vi "SA Configure.vi"(7 "RBW(Hz)":dbl=1.0, 8 "number of records":dbl=1.0, 9 "samples per record":dbl=100.0, 10 "IQ Rate (S/s)":dbl=4000000.0 format="%#.3p", 11 "Semiconductor Module Context":T1) -> (0 "error out":errorcluster)   [LabVIEW 2014]
uses:
  <vilib>/NI_TestStand_SemiconductorModule/NI_TestStand_Semiconductor_Module.lvlibp/PinMap/General/SemiconductorModuleContext.ctl
  <instrlib>/niRFSA/niRFSA.llb/niRFSA Acquisition Types.ctl
  <vilib>/NI_TestStand_SemiconductorModule/NI_TestStand_Semiconductor_Module.lvlibp
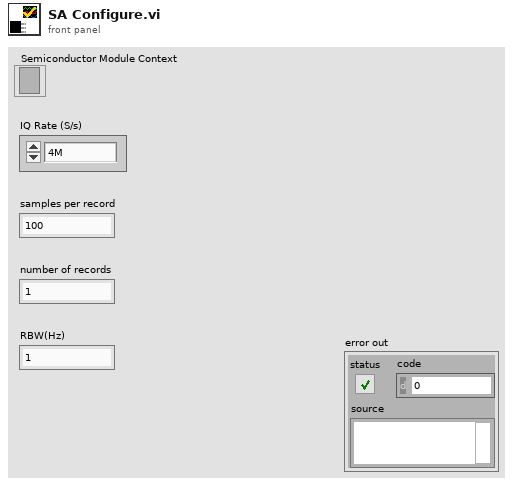
[diagram p1: front panel]
types:
  T1 = typedef "NI_TestStand_Semiconductor_Module.lvlibp/SemiconductorModuleContext.ctl" = refnum<k7>
  T2 = typedef "niRFSA Acquisition Types.ctl" = i32
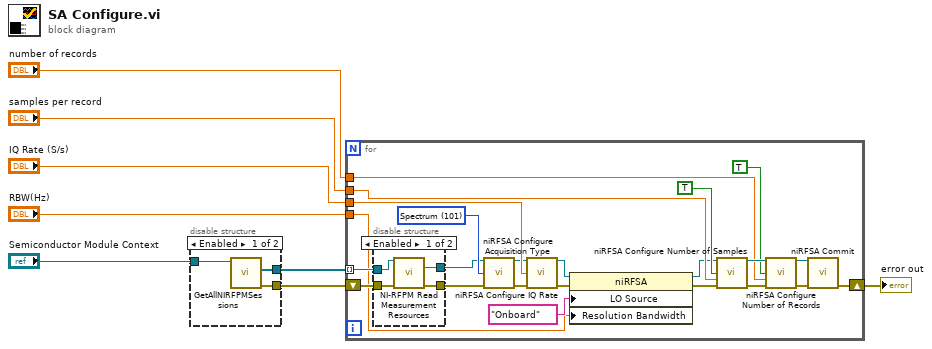
[diagram p0: block diagram]
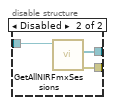
[diagram p2: hidden frame]
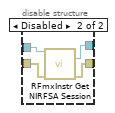
[diagram p3: hidden frame]
diagram:
  n1 = disable-structure shown="Enabled" {
    disable-tunnel: [w11 w13] -> w8
    disable-tunnel: "Semiconductor Module Context" -> [w10 w14]
    disable-tunnel: [w9 w12] -> w6
    frame Enabled {
      n2 = call <vilib>:"GetAllNIRFPMSessions.vi"("Semiconductor Module Context"=w10) -> ("error out"=w11:errorcluster, "Instrument Sessions"=w9:refnum<k15>[])  [unwired: 8 in, 1 out]
    }
    frame Disabled {
      n3 = call <vilib>:"GetAllNIRFmxSessions.vi"("Semiconductor Module Context"=w14) -> ("error out"=w13:errorcluster, "Instrument Sessions"=w12:refnum<k21>[])  [unwired: 8 in, 1 out]
    }
  }
  n4 = for {
    shift-right: [w27] -> w2
    shift-left: w8 -> [w18]
    tunnel: w6 -> [w19] mode=indexing
    tunnel: "IQ Rate (S/s)" -> [w36]
    tunnel: "samples per record" -> [w31]
    tunnel: "number of records" -> [w30]
    tunnel: "RBW(Hz)" -> [w15]
    w37 = T2 101 items=["IQ"=100, "Spectrum"=101] ("acquisition type")
    n5 = disable-structure shown="Enabled" {
      disable-tunnel: w19 -> [w41 w45]
      disable-tunnel: w18 -> [w40 w43]
      disable-tunnel: [w39 w44] -> w17
      disable-tunnel: [w38 w42] -> w16
      frame Enabled {
        n6 = call <instrlib>:"NI-RFPM Read Measurement Resources.vi"("NI-5530 handle in"=w41, "error in"=w40) -> ("RFSA handle"=w39:refnum<k15>, "error out"=w38:errorcluster)  [unwired: 9 in, 3 out]
      }
      frame Disabled {
        n7 = call <vilib>:"RFmxInstr Get NIRFSA Session.vi"("Instrument Handle In"=w45, "error in (no error)"=w43) -> ("NI RFSA Session"=w44:refnum<k15>, "error out"=w42:errorcluster)  [unwired: 11 in, 1 out]
      }
    }
    n8 = call <instrlib>:"niRFSA Configure Acquisition Type.vi"("instrument handle"=w17, "acquisition type"=w37, "error in"=w16) -> ("instrument handle out"=w21:refnum<k15>, "error out"=w20:errorcluster)  [unwired: 11 in]
    n9 = call <instrlib>:"niRFSA Configure IQ Rate.vi"("instrument handle"=w21, "IQ rate (S/s)"=w36, "error in"=w20) -> ("instrument handle out"=w26:refnum<k15>, "error out"=w24:errorcluster)  [unwired: 11 in]
    n10 = property class="niRFSA"(reference=w26, error in=w24, "LO Source"="Onboard" ("Signal Path:LO Source"), "Resolution Bandwidth"=w15) -> (reference out=w25:refnum<k15>, error out=w23:errorcluster)
    n11 = call <instrlib>:"niRFSA Configure Number of Samples.vi"("instrument handle"=w25, "number of samples is finite"=TRUE, "samples per record"=w31, "error in"=w23) -> ("instrument handle out"=w34:refnum<k15>, "error out"=w35:errorcluster)  [unwired: 10 in]
    n12 = call <instrlib>:"niRFSA Configure Number of Records.vi"("instrument handle"=w34, "number of records is finite"=TRUE, "number of records"=w30, "error in"=w35) -> ("instrument handle out"=w28:refnum<k15>, "error out"=w29:errorcluster)  [unwired: 10 in]
    n13 = call <instrlib>:"niRFSA Commit.vi"("instrument handle"=w28, "error in"=w29) -> ("error out"=w27:errorcluster)  [unwired: 12 in, 1 out]
  }
  "error out" <- w2
